vi "2023 InitGlobalConstants.vi"(1 "error in (no error)":errorcluster, 2 "localConstantSpreadSheet":string[][](array[string])) -> (0 "error out":errorcluster)   [LabVIEW 2020]
uses:
  <vilib>/Rock Robotics/WPI/ThirdParty/Phoenix-LabVIEW/Motor Controller/Controls/CTRE_Phoenix_MotorControl_ControlMode.ctl
  2023 Robot Global Data.vi
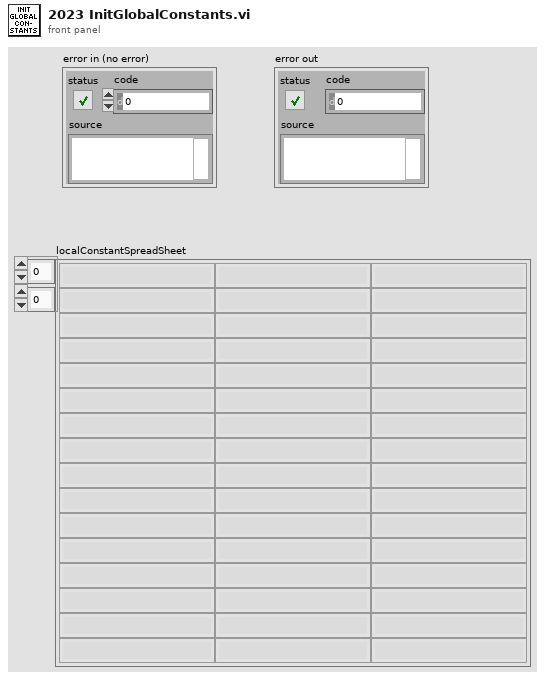
[diagram p1: front panel]
types:
  T1 = typedef "CTRE_Phoenix_MotorControl_ControlMode.ctl" = u16
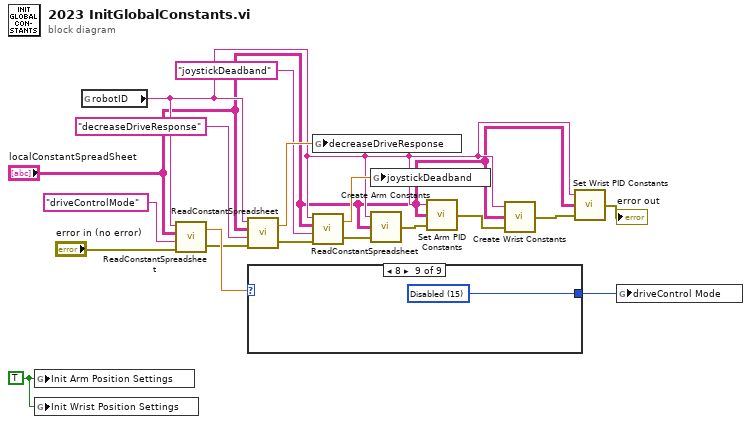
[diagram p0: block diagram]
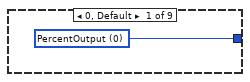
[diagram p2: hidden frame]
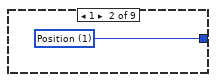
[diagram p3: hidden frame]
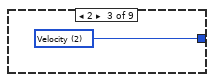
[diagram p4: hidden frame]
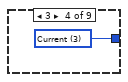
[diagram p5: hidden frame]
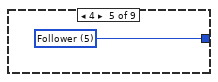
[diagram p6: hidden frame]
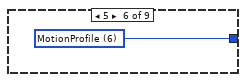
[diagram p7: hidden frame]
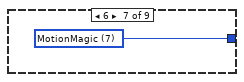
[diagram p8: hidden frame]
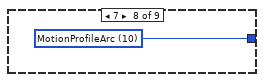
[diagram p9: hidden frame]
diagram:
  w5 = TRUE ("First Time")
  n1 = global write "2023 Robot Global Data.vi" "Init Arm Position Settings"(w5) -> ()
  n2 = global write "2023 Robot Global Data.vi" "Init Wrist Position Settings"(w5) -> ()
  n3 = global read "2023 Robot Global Data.vi" "robotID"() -> (w4:string)
  n4 = call "ReadConstantSpreadsheet.vi"("error in"="error in (no error)", "Constant"="driveControlMode", "2023ConstantSpreadSheet"="localConstantSpreadSheet", "Robot ID"=w4) -> ("error out"=w12:errorcluster, "Constant Value"=w17:dbl)
  n5 = call "ReadConstantSpreadsheet.vi"("error in"=w12, "Constant"="decreaseDriveResponse", "2023ConstantSpreadSheet"="localConstantSpreadSheet", "Robot ID"=w4) -> ("error out"=w10:errorcluster, "Constant Value"=w14:dbl)
  n6 = case shown="8" w17 {
    tunnel: [w19 w20 w21 w22 w23 w24 w25 w26 w27] -> w15
    frame 0, Default {
      w19 = T1 0 items=["PercentOutput"=0, "Position"=1, "Velocity"=2, "Current"=3, "Follower"=5, "MotionProfile"=6, "MotionMagic"=7, "MotionProfileArc"=10, "Disabled"=15] ("driveControl Mode")
    }
    frame 1 {
      w20 = T1 1 items=["PercentOutput"=0, "Position"=1, "Velocity"=2, "Current"=3, "Follower"=5, "MotionProfile"=6, "MotionMagic"=7, "MotionProfileArc"=10, "Disabled"=15] ("driveControl Mode")
    }
    frame 2 {
      w21 = T1 2 items=["PercentOutput"=0, "Position"=1, "Velocity"=2, "Current"=3, "Follower"=5, "MotionProfile"=6, "MotionMagic"=7, "MotionProfileArc"=10, "Disabled"=15] ("driveControl Mode")
    }
    frame 3 {
      w22 = T1 3 items=["PercentOutput"=0, "Position"=1, "Velocity"=2, "Current"=3, "Follower"=5, "MotionProfile"=6, "MotionMagic"=7, "MotionProfileArc"=10, "Disabled"=15] ("driveControl Mode")
    }
    frame 4 {
      w23 = T1 5 items=["PercentOutput"=0, "Position"=1, "Velocity"=2, "Current"=3, "Follower"=5, "MotionProfile"=6, "MotionMagic"=7, "MotionProfileArc"=10, "Disabled"=15] ("driveControl Mode")
    }
    frame 5 {
      w24 = T1 6 items=["PercentOutput"=0, "Position"=1, "Velocity"=2, "Current"=3, "Follower"=5, "MotionProfile"=6, "MotionMagic"=7, "MotionProfileArc"=10, "Disabled"=15] ("driveControl Mode")
    }
    frame 6 {
      w25 = T1 7 items=["PercentOutput"=0, "Position"=1, "Velocity"=2, "Current"=3, "Follower"=5, "MotionProfile"=6, "MotionMagic"=7, "MotionProfileArc"=10, "Disabled"=15] ("driveControl Mode")
    }
    frame 7 {
      w26 = T1 10 items=["PercentOutput"=0, "Position"=1, "Velocity"=2, "Current"=3, "Follower"=5, "MotionProfile"=6, "MotionMagic"=7, "MotionProfileArc"=10, "Disabled"=15] ("driveControl Mode")
    }
    frame 8 {
      w27 = T1 15 items=["PercentOutput"=0, "Position"=1, "Velocity"=2, "Current"=3, "Follower"=5, "MotionProfile"=6, "MotionMagic"=7, "MotionProfileArc"=10, "Disabled"=15] ("driveControl Mode")
    }
  }
  n7 = global write "2023 Robot Global Data.vi" "decreaseDriveResponse"(w14) -> ()
  n8 = call "ReadConstantSpreadsheet.vi"("error in"=w10, "Constant"="joystickDeadband", "2023ConstantSpreadSheet"="localConstantSpreadSheet", "Robot ID"=w4) -> ("error out"=w9:errorcluster, "Constant Value"=w7:dbl)
  n9 = global write "2023 Robot Global Data.vi" "joystickDeadband"(w7) -> ()
  n10 = call "Create Arm Constants.vi"("error in"=w9, "localConstantSpreadSheet"="localConstantSpreadSheet", "robotID"=w4) -> ("error out"=w11:errorcluster)
  n11 = call "Set Arm PID Constants.vi"("error in (no error)"=w11, "localConstantSpreadSheet"="localConstantSpreadSheet", "robotID"=w4) -> ("error out"=w6:errorcluster)
  n12 = call "Create Wrist Constants.vi"("error in"=w6, "localConstantSpreadSheet"="localConstantSpreadSheet", "robotID"=w4) -> ("error out"=w2:errorcluster)
  n13 = call "Set Wrist PID Constants.vi"("error in (no error)"=w2, "localConstantSpreadSheet"="localConstantSpreadSheet", "robotID"=w4) -> ("error out"=→"error out":errorcluster)
  n14 = global write "2023 Robot Global Data.vi" "driveControl Mode"(w15) -> ()
